vi "Check Condition.vi"(8 "error in (no error)":errorcluster, 10 "Expression Data":T1, 11 "Output Sequencer in":refnum<class "Output Sequencer.lvclass">) -> (0 "error out":errorcluster, 1 "Condition empty":bool, 2 "Check passed":bool, 3 "Output Sequencer out":refnum<class "Output Sequencer.lvclass">)   [LabVIEW 2020, in "Output Sequencer.lvlib" / "Output Sequencer.lvclass"]
uses:
  Output Sequencer.lvclass
  Types/Expression Data.ctl
  <vilib>/LAVA/muParser/mupExpr/mupExpr.lvclass
  <vilib>/LAVA/muParser/mupExpr/mupExpr.lvclass/mupExpr.ctl
  <vilib>/LAVA/muParser/mupExpr/Eval_MultiVar_SglRes.vi
  <vilib>/LAVA/muParser/mupExpr/SetVarVal.vi
  <vilib>/LAVA/muParser/mupLib/mupEval.vi
  <vilib>/LAVA/muParser/mupLib/mupSetVarValue.vi
  <vilib>/LAVA/muParser/mupLib/mupCheckError.vi
  <vilib>/Utility/error.llb/Error Cluster From Error Code.vi
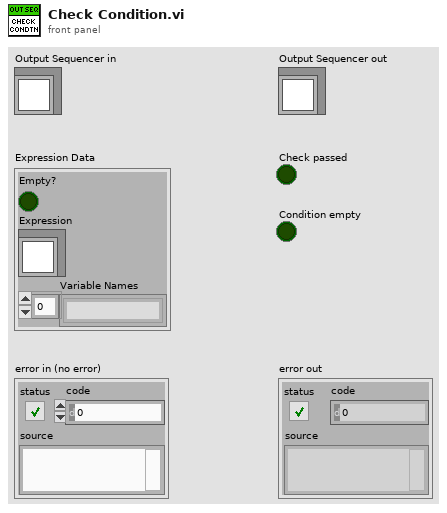
[diagram p1: front panel]
types:
  T1 = typedef "Output Sequencer.lvlib/Output Sequencer.lvclass/Expression Data.ctl" = cluster{"Empty?":bool, "Expression":refnum<class "mupExpr.lvclass">, "Variable Names":string[]}
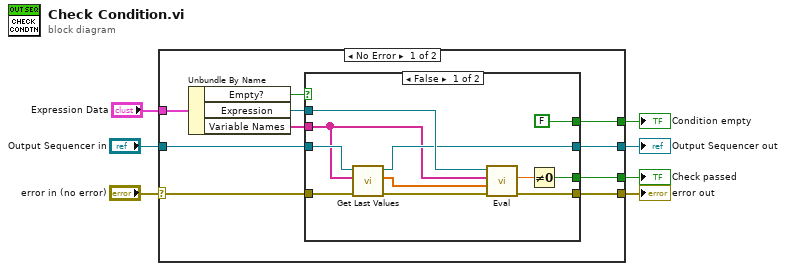
[diagram p0: block diagram]
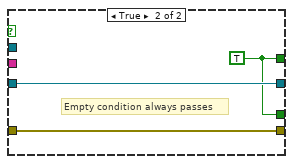
[diagram p2: hidden frame]
diagram:
  n1 = case shown="No Error" "error in (no error)" {
    selector: "error in (no error)" -> [w8 w33]
    tunnel: [w17 _] -> w7
    tunnel: [w16 w32] -> w6
    tunnel: "Output Sequencer in" -> [w15 w32]
    tunnel: [w14 _] -> w4
    tunnel: "Expression Data" -> [w13 _]
    tunnel: [w9 w33] -> w2
    frame No Error {
      n2 = Unbundle By Name(w13) -> ("Empty?"=w12:bool, "Expression"=w11:refnum<class "mupExpr.lvclass">, "Variable Names"=w10:string[])
      n3 = case shown="False" w12 {
        tunnel: w11 -> [w28 _]
        tunnel: w10 -> [w24 _]
        tunnel: w15 -> [w27 w31]
        tunnel: [w26 w31] -> w16
        tunnel: [w21 w30] -> w17
        tunnel: [FALSE w30] -> w14
        tunnel: w8 -> [w20 w29]
        tunnel: [w18 w29] -> w9
        frame False {
          n4 = call "Get Last Values.vi"("error in (no error)"=w20, "Variables"=w24, "Output Sequencer in"=w27) -> ("error out"=w19:errorcluster, "Values"=w23:dbl[], "Output Sequencer out"=w26:refnum<class "Output Sequencer.lvclass">)  [unwired: 6 in]
          n5 = call-poly <vilib>:"Eval.vi"("error in (no error)"=w19, "varValues"=w23, "varNames"=w24, "muExpr in"=w28) -> ("error out"=w18:errorcluster, "Result"=w22:dbl)  [unwired: 5 in, 1 out]
          n6 = Not Equal To 0?(x=w22) -> (x != 0?=w21:bool)
        }
        frame True {
          w30 = TRUE
          # "Empty condition always passes"
        }
      }
    }
    frame Error {
    }
  }
  "Check passed" <- w7
  "Output Sequencer out" <- w6
  "Condition empty" <- w4
  "error out" <- w2
